vi "GetDateHour.vi"() -> (6 "Date":string, 8 "Hour":string)   [LabVIEW 2023]
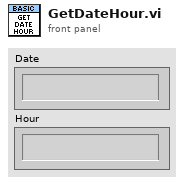
[diagram p1: front panel]
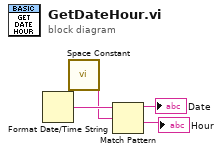
[diagram p0: block diagram]
diagram:
  n1 = Format Date/Time String() -> (date/time string=w4:string)  [unwired: 3 in]
  n2 = call <vilib>:"Space Constant.vi"() -> ("String"=w3:string)
  n3 = Match Pattern(string=w4, regular expression=w3) -> (before substring=→"Date":string, after substring=→"Hour":string)  [unwired: 1 in, 2 out]
